vi "EXCOM_28.vi"(0 "VRN IN":refnum<visa-resource-name>) -> (2 "RA":dbl format="%.8f", 3 "DEC":dbl format="%.8f", 4 "VRN OUT":refnum<visa-resource-name>, 8 "OK Done":bool, 13 "RAadj":dbl format="%.8f", 14 "DECadj":dbl format="%.8f", 15 "error out":errorcluster)   [LabVIEW 2010]
panel:
  # "3 = COM4"
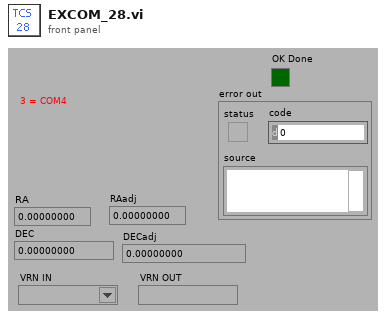
[diagram p1: front panel]
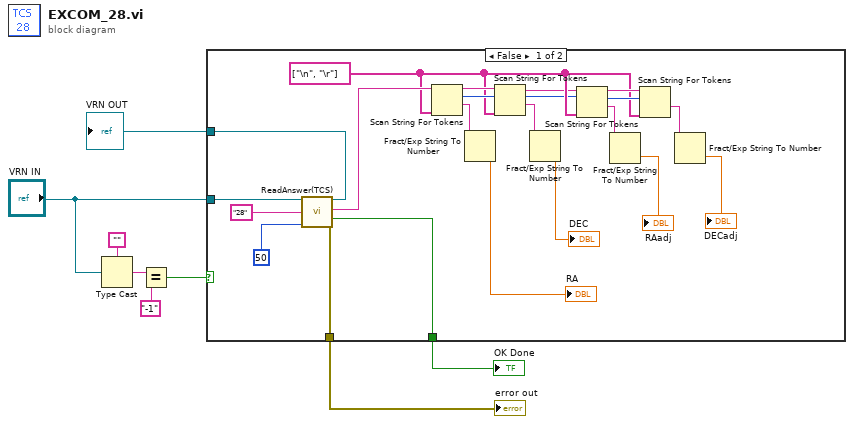
[diagram p0: block diagram]
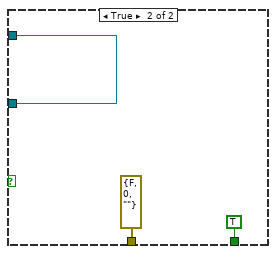
[diagram p2: hidden frame]
diagram:
  n1 = Type Cast(type="", x="VRN IN") -> (*(type *) &x=w6:string)
  n2 = Equal?(x=w6, y="-1") -> (x = y?=w3:bool)
  n3 = case shown="False" w3 {
    tunnel: [w27 TRUE ("OK Done")] -> w8
    tunnel: "VRN IN" -> [w11 w31]
    tunnel: [w10 errorcluster {"status"=FALSE, "code"=0, "source"=""} ("error out")] -> w2
    tunnel: [w9 w31] -> w1
    frame False {
      w16 = string[] ["\n", "\r"] ("delimiters (\\s,\\t,\\r,\\n)")
      n4 = call "ReadAnswer(TCS).vi"("VISA resource name"=w11, "String to Send"="28", "Bytes to Read"=u32 50) -> ("VISA resource name dup"=w9:refnum<visa-resource-name>, "String Received"=w23:string, "OK Done"=w27:bool, "error out"=w10:errorcluster)  [unwired: 9 in]
      n5 = Scan String For Tokens(6:w16, 9:w23) -> (1:w25:string, 2:w29:i32, 3:w28:string)  [unwired: 4 in, 1 out]
      n6 = Fract/Exp String To Number(string=w25) -> (number=→"RA":dbl)  [unwired: 3 in, 1 out]
      n7 = Scan String For Tokens(6:w16, 8:w29, 9:w28) -> (1:w26:string, 2:w12:i32, 3:w15:string)  [unwired: 3 in, 1 out]
      n8 = Fract/Exp String To Number(string=w26) -> (number=→"DEC":dbl)  [unwired: 3 in, 1 out]
      n9 = Scan String For Tokens(6:w16, 8:w12, 9:w15) -> (1:w20:string, 2:w17:i32, 3:w18:string)  [unwired: 3 in, 1 out]
      n10 = Fract/Exp String To Number(string=w20) -> (number=→"RAadj":dbl)  [unwired: 3 in, 1 out]
      n11 = Scan String For Tokens(6:w16, 8:w17, 9:w18) -> (1:w19:string)  [unwired: 3 in, 3 out]
      n12 = Fract/Exp String To Number(string=w19) -> (number=→"DECadj":dbl)  [unwired: 3 in, 1 out]
    }
    frame True {
    }
  }
  "OK Done" <- w8
  "error out" <- w2
  "VRN OUT" <- w1
